vi "Const Temp Coordinate 2 points.vi"() -> (3 "Const Temp Coordinate":T1={"Horizontal"=-10000, "Vertical"=-10000})   [LabVIEW 2021]
uses:
  <vilib>/Utility/miscctls.llb/LVPoint32TypeDef.ctl
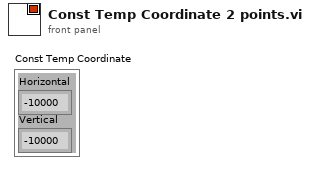
[diagram p1: front panel]
types:
  T1 = typedef "LVPoint32TypeDef.ctl" = cluster{"Horizontal":i32, "Vertical":i32}
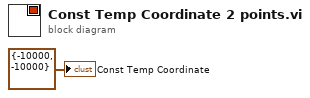
[diagram p0: block diagram]
diagram:
  "Const Temp Coordinate" <- T1 {"Horizontal"=-10000, "Vertical"=-10000} ("Temp Coord")
